vi "Get timestamp.vi"(8 "error in (no error)":errorcluster) -> (0 "error out":errorcluster, 1 "time string":string, 2 "date string":string, 3 "Timestamp":string, 4 "Timestamp msec":string, 5 "date_underscore":string, 6 "time_underscore":string, 7 "Date_time_for_filenames":string, 11 "Year last 2 digits":string)   [LabVIEW 2024]
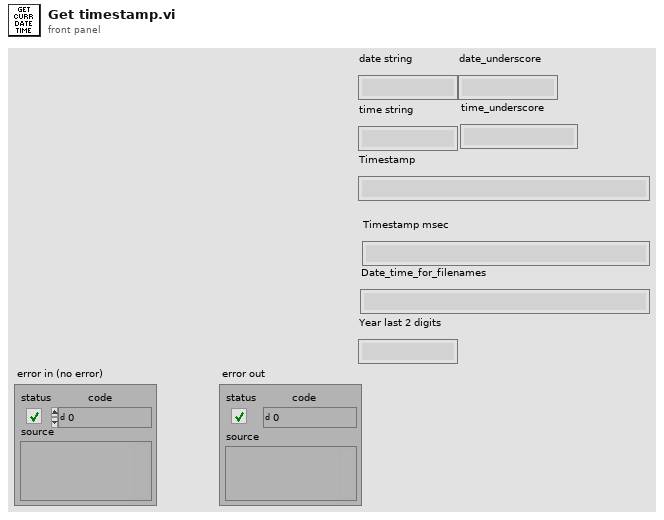
[diagram p1: front panel]
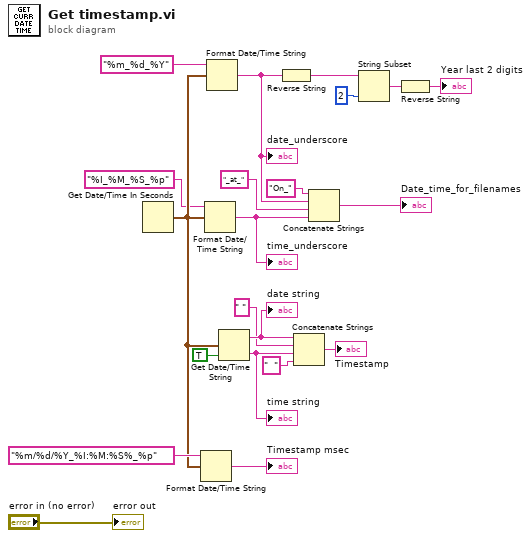
[diagram p0: block diagram]
diagram:
  n1 = Get Date/Time In Seconds() -> (seconds since 1Jan1904=w12:timestamp)
  n2 = Format Date/Time String(time format string (%c)="%m/%d/%Y_%I:%M:%S%_%p", seconds (now)=w12) -> (date/time string=→"Timestamp msec":string)  [unwired: 1 in]
  n3 = Format Date/Time String(time format string (%c)="%I_%M_%S_%p", seconds (now)=w12) -> (date/time string=w7:string)  [unwired: 1 in]
  "time_underscore" <- w7
  n4 = Format Date/Time String(time format string (%c)="%m_%d_%Y", seconds (now)=w12) -> (date/time string=w5:string)  [unwired: 1 in]
  "date_underscore" <- w5
  n5 = Get Date/Time String(seconds (now)=w12, want seconds? (F)=TRUE) -> (date string=w19:string, time string=w17:string)  [unwired: 1 in]
  "date string" <- w19
  "time string" <- w17
  n6 = Reverse String(1:w5) -> (0:w4:string)
  n7 = Concatenate Strings(w19, " " ("string"), w17, "  " ("string")) -> (→"Timestamp":string)
  n8 = Concatenate Strings("On_" ("string"), w5, "_at_" ("string"), w7) -> (→"Date_time_for_filenames":string)
  n9 = String Subset(string=w4, length (rest)=2 ("length (rest)")) -> (substring=w2:string)  [unwired: 1 in]
  n10 = Reverse String(1:w2) -> (0:→"Year last 2 digits":string)
  "error out" <- "error in (no error)"
